vi "APC_9049_SparkSettings.vi"(1 "MAX_CAT":u16=28400, 2 "CutoffPosition (DBTDC)":sgl=-180.0, 3 "SparkTiming (DBTDC) loc":sgl, 4 "TDC (Absolute CAD)":sgl, 5 "SparkEnable":bool) -> (0 "SparkControl":T1)   [LabVIEW 2020]
doc: "This example demonstrates the procedure required to apply different NI-DAQmx Custom Scales to each virtual channel in a task. A DAQmx Task Property Node (Functions >> NI Measurements >> DAQmx - Data Acquisition >> DAQmx Advanced Task Options) is used to obtain the task's virtual channels. A DAQmx Channel Property Node (Functions >> NI Measurements >> DAQmx - Data Acquisition) is then used to set the custom scale for each virtual channel in the task.\n\nThe \"DAQmx Create Scale\" VI creates a custom scale for each channel in the channel list. *Note, make sure your Minimum and Maximum channel parameters are consistent with the range the scale will create."
panel:
  in  "MaxDwell (msec)":sgl=6.0
  in  "MinDwell (msec)":sgl=2.0
  in  "Dwell (msec)":sgl=4.0
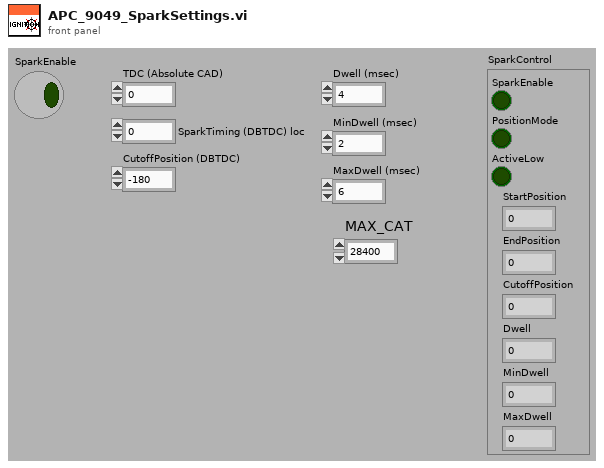
[diagram p1: front panel]
types:
  T1 = cluster{"SparkEnable":bool, "PositionMode":bool, "ActiveLow":bool, "StartPosition":u16, "EndPosition":u16, "CutoffPosition":u16, "Dwell":u32, "MinDwell":u32, "MaxDwell":u32}
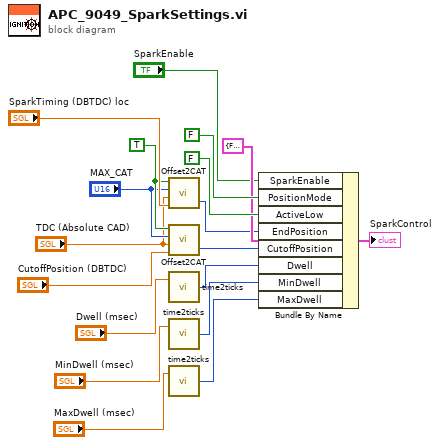
[diagram p0: block diagram]
diagram:
  w6 = TRUE ("Stroke (FALSE=2, TRUE=4)")
  n1 = call <vilib>:"Offset2CAT.vi"("Offset (CAD Before TDC)"="SparkTiming (DBTDC) loc", "TDC (Absolute CAD)"="TDC (Absolute CAD)", "MAX_CAT"="MAX_CAT", "Stroke (FALSE=2, TRUE=4)"=w6) -> ("CAT"=w7:u16)  [unwired: 1 out]
  n2 = call <vilib>:"Offset2CAT.vi"("Offset (CAD Before TDC)"="CutoffPosition (DBTDC)", "TDC (Absolute CAD)"="TDC (Absolute CAD)", "MAX_CAT"="MAX_CAT", "Stroke (FALSE=2, TRUE=4)"=w6) -> ("CAT"=w4:u16)  [unwired: 1 out]
  n3 = call <vilib>:"time2ticks.vi"("Time (msec)"="Dwell (msec)") -> ("Ticks"=w13:u32)  [unwired: 1 in]
  n4 = call <vilib>:"time2ticks.vi"("Time (msec)"="MinDwell (msec)") -> ("Ticks"=w12:u32)  [unwired: 1 in]
  n5 = call <vilib>:"time2ticks.vi"("Time (msec)"="MaxDwell (msec)") -> ("Ticks"=w11:u32)  [unwired: 1 in]
  n6 = Bundle By Name(cluster=T1 {"SparkEnable"=FALSE, "PositionMode"=FALSE, "ActiveLow"=FALSE, "StartPosition"=0, "EndPosition"=0, "CutoffPosition"=0, "Dwell"=0, "MinDwell"=0, "MaxDwell"=0} ("SparkControl"), "SparkEnable"="SparkEnable", "PositionMode"=FALSE, "ActiveLow"=FALSE, "EndPosition"=w7, "CutoffPosition"=w4, "Dwell"=w13, "MinDwell"=w12, "MaxDwell"=w11) -> (→"SparkControl":T1)
